vi "high_field_probe_peaks.vi"() -> ()   [LabVIEW 2011]
uses:
  <vilib>/express/express arith-compare/Formula/XNode/ExpressFormulaBlockNode.xnode
  <vilib>/Analysis/NI_AAL_SigProc.lvlib
panel:
  in  "peak threshold":dbl=0.01 format="%0.2f"
  out "Amplitudes":dbl[](array[numeric])
  in  "Fits?":bool
  out "Waveform Chart 2":dbl(graph)
  out "best fit parameters":dbl[](array[numeric])
  in  "Set Zero Peaks":bool
  out "Peak 2 Amp":dbl
  out "Peak 1 Amp":dbl
  out "Polarization":dbl
  out "Peak Ratio":dbl
  out "XY Graph":cluster{dbl[], dbl[]}[](graph)
  in  "Peak 2 at Zero":dbl=1.0
  in  "Peak 1 at Zero":dbl=1.0
  in  "fit parameters":dbl[](array[numeric])=[0.04, 0.4, 0.12, 0.03, 0.8, 0.15, 0.06, 1.4, 0.15]
  in  "stop":bool
  in  "Center Freq":dbl=400.0
  in  "Voltage Sweep Range":i32=2
  out "Current Set Voltage":dbl
  in  "threshold":dbl=0.01
  in  "rate":dbl=4000.0
  in  "number of samples":i32=100
  out "data":dynamicdata(graph)
  out "Waveform Chart":dbl(graph)
  out "amplitude":dbl
  out "frequency":dbl
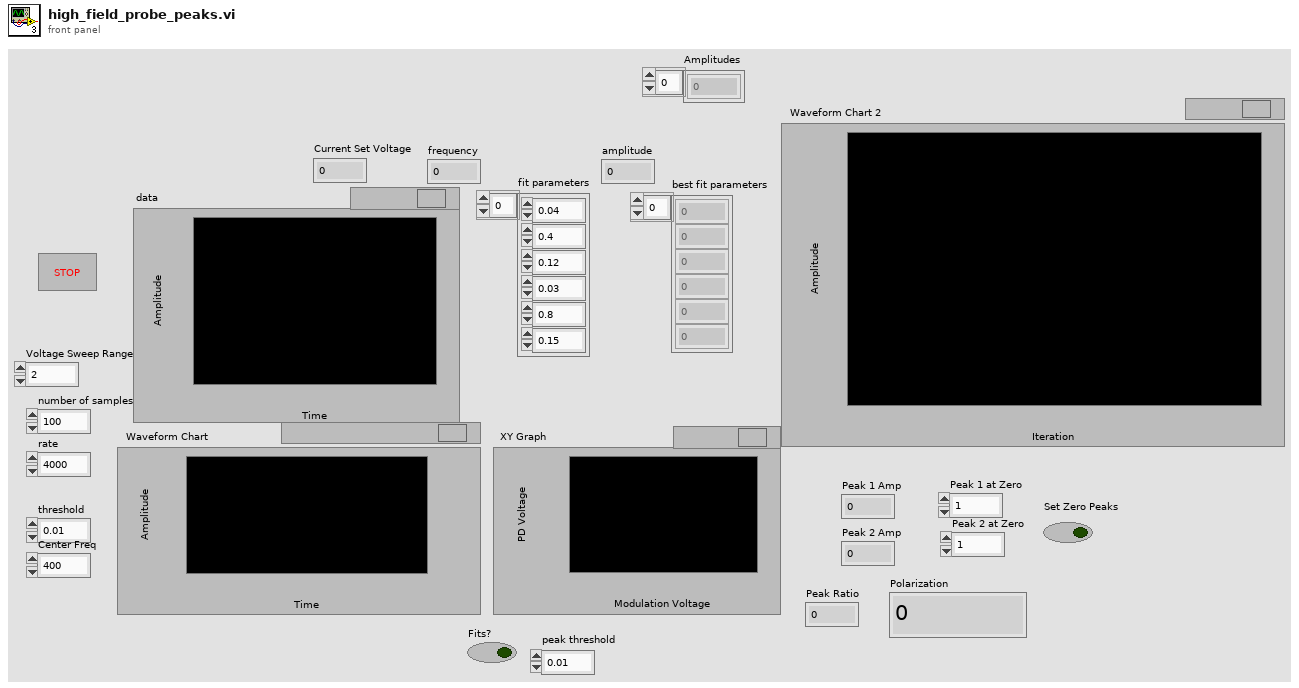
[diagram p1: front panel]
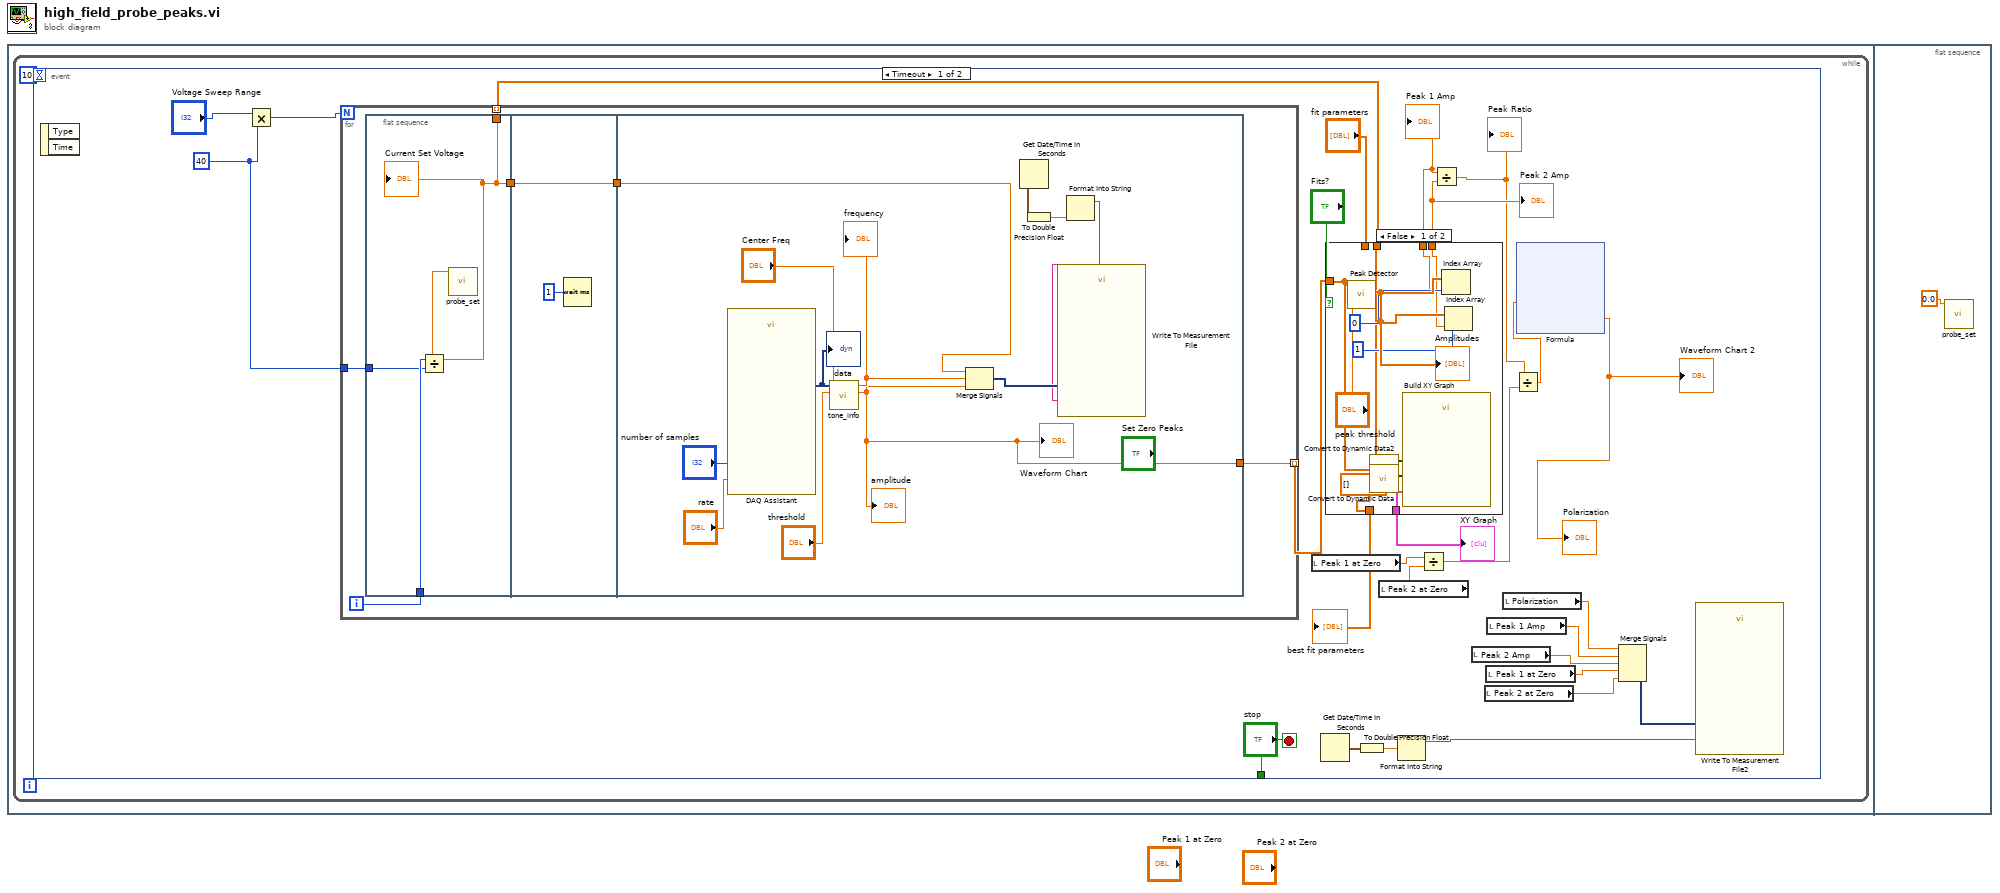
[diagram p0: block diagram]
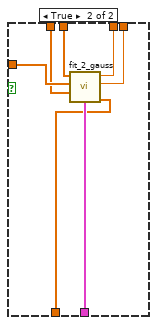
[diagram p2: hidden frame]
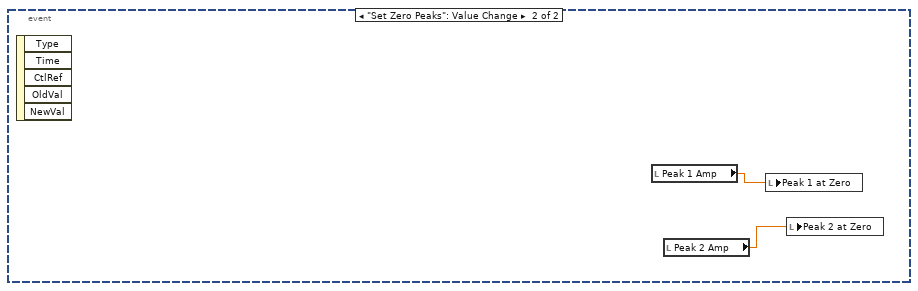
[diagram p3: hidden frame]
diagram:
  n1 = flat-sequence {
    frame #0 {
      n2 = while {
        stop <- w2 stop-if-true
        n3 = event shown="[0] Timeout" {
          selector: _ -> [_ _]
          dyn-events: _ -> [_ _]
          timeout: 10 -> [_ _]
          tunnel: ["stop" _] -> w2
          event Timeout {
            w27 = 40 ("y")
            n4 = event-data() -> ()  [unwired: 1 in, 2 out]
            n5 = Multiply(x="Voltage Sweep Range", y=w27) -> (x*y=w28:i32)
            n6 = for {
              N: w28 -> [_]
              tunnel: w27 -> [w61]
              tunnel: [w58] -> w25 mode=indexing
              tunnel: [w57] -> w23 mode=indexing
              i -> [w62]
              n7 = flat-sequence {
                tunnel: w62 -> [w65]
                tunnel: w61 -> [w64]
                tunnel: [w63] -> w59
                tunnel: [w63] -> w57
                tunnel: [w66] -> w60
                tunnel: w59 -> [w66]
                tunnel: w60 -> [w72]
                tunnel: [w68] -> w58
                frame #0 {
                  n8 = Divide(x=w65, y=w64) -> (x/y=w63:dbl)
                  "Current Set Voltage" <- w63
                  n9 = call "probe_set.vi"("Voltage"=w63) -> ()  [unwired: 11 in]
                }
                frame #1 {
                  n10 = Wait (ms)(milliseconds to wait=u32 1) -> ()  [unwired: 1 out]
                }
                frame #2 {
                  n11 = call "DAQ Assistant"("rate"="rate", "number of samples"="number of samples") -> ("data"=w75:dynamicdata)  [unwired: 15 in, 2 out]
                  "data" <- w75
                  n12 = call "tone_info.vi"("Center Freq"="Center Freq", "threshold"="threshold", "time signal in"=w75) -> ("amplitude"=w68:dbl, "frequency"=w79:dbl)  [unwired: 6 in, 1 out]
                  "frequency" <- w79
                  "amplitude" <- w68
                  "Waveform Chart" <- w68
                  n13 = Merge Signals(w72, w79, w68) -> (w74:dynamicdata)
                  n14 = Get Date/Time In Seconds() -> (seconds since 1Jan1904=w71:timestamp)
                  n15 = To Double Precision Float(number=w71) -> (double precision float=w70:dbl)
                  n16 = Format Into String(w70) -> (resulting string=w69:string)  [unwired: 3 in, 1 out]
                  n17 = call "Write To Measurement File"("Signals"=w74, "Comment"=w69) -> ()  [unwired: 15 in, 3 out]
                }
              }
            }
            n18 = local read "Peak 1 at Zero"() -> (w15:dbl)
            n19 = Get Date/Time In Seconds() -> (seconds since 1Jan1904=w12:timestamp)
            n20 = case shown="False" "Fits?" {
              tunnel: w25 -> [w35 w48]
              tunnel: "fit parameters" -> [_ w47]
              tunnel: w23 -> [w33 w46]
              tunnel: [w37 w45] -> w22
              tunnel: [w36 w44] -> w21
              tunnel: [w31 w43] -> w20
              tunnel: [dbl[] [] ("best fit parameters") w42] -> w10
              frame False {
                n21 = call <vilib>:"Peak Detector.vi"("threshold"="peak threshold", "X"=w35) -> ("Amplitudes"=w40:dbl[])  [unwired: 5 in, 4 out]
                "Amplitudes" <- w40
                n22 = call "Convert to Dynamic Data2"("Array"=w33) -> ("Dynamic Data Type"=w32:dynamicdata)  [unwired: 3 in]
                n23 = call "Convert to Dynamic Data"("Array"=w35) -> ("Dynamic Data Type"=w34:dynamicdata)  [unwired: 3 in]
                n24 = call "Build XY Graph"("Y Input"=w34, "X Input"=w32) -> ("XY Graph"=w31:cluster{"Y":dbl[], "Y":dbl[]}[])  [unwired: 3 in, 6 out]
                n25 = Index Array(array=w40, index=0) -> (element=w37:dbl)
                n26 = Index Array(array=w40, index=1) -> (element=w36:dbl)
              }
              frame True {
                n27 = call "fit_2_gauss.vi"("initial parameters"=w47, "y Array"=w48, "x Array"=w46) -> ("best fit parameters"=w42:dbl[], "XY Graph"=w43:cluster{dbl[], dbl[]}[], "Peak 2 Amp"=w44:dbl, "Peak 1 Amp"=w45:dbl)  [unwired: 5 in]
              }
            }
            "XY Graph" <- w20
            "Peak 1 Amp" <- w22
            "Peak 2 Amp" <- w21
            "best fit parameters" <- w10
            n28 = To Double Precision Float(number=w12) -> (double precision float=w11:dbl)
            n29 = local read "Peak 2 at Zero"() -> (w14:dbl)
            n30 = Format Into String(w11) -> (resulting string=w19:string)  [unwired: 3 in, 1 out]
            n31 = Divide(x=w15, y=w14) -> (x/y=w17:dbl)
            n32 = Divide(x=w22, y=w21) -> (x/y=w18:dbl)
            "Peak Ratio" <- w18
            n33 = local read "Peak 2 Amp"() -> (w6:dbl)
            n34 = local read "Peak 2 at Zero"() -> (w4:dbl)
            n35 = local read "Peak 1 at Zero"() -> (w5:dbl)
            n36 = local read "Peak 1 Amp"() -> (w7:dbl)
            n37 = local read "Polarization"() -> (w8:dbl)
            n38 = Divide(x=w18, y=w17) -> (x/y=w16:dbl)
            n39 = xnode "Formula"("X"=w16) -> ("Result"=→"Polarization" →"Waveform Chart 2":dbl)  [unwired: 1 in, 1 out]
            n40 = Merge Signals(w8, w7, w6, w5, w4) -> (w13:dynamicdata)
            n41 = call "Write To Measurement File2"("Signals"=w13, "Comment"=w19) -> ()  [unwired: 15 in, 3 out]
          }
          event "Set Zero Peaks": Value Change {
            n42 = event-data() -> ()  [unwired: 1 in, 5 out]
            n43 = local read "Peak 1 Amp"() -> (w81:dbl)
            n44 = local read "Peak 2 Amp"() -> (w80:dbl)
            n45 = local write "Peak 1 at Zero"(w81) -> ()
            n46 = local write "Peak 2 at Zero"(w80) -> ()
          }
        }
      }
    }
    frame #1 {
      n47 = call "probe_set.vi"("Voltage"=0.0) -> ()  [unwired: 11 in]
    }
  }
